vi "Read_CAL_PARAMETER_Connector_A.vi"() -> ()   [LabVIEW 2016]
doc: "The myRIO Project template acquires acceleration data from the onboard accelerometer and displays the changes of acceleration values in a waveform chart."
panel:
  in  "Tab Control":T1(tab)
  out "Device_ID 2":u8[](array[numeric]) format="%.0x"
  out "READ LSB CAL_PARAM 2":u8[][](array[numeric]) format="%.0x"
  out "READ MSB CAL_PARAM 2":u8[][](array[numeric]) format="%.0x"
  out "Array 3":i16[][](array[numeric])
  out "UT_Value 2":u16[](array[numeric])
  out "Temperature(°C)":dbl
  out "Waveform Chart Temperature":dbl(graph)
  out "Waveform Chart Presssure":dbl(graph)
  out "Pressure in Pa.":dbl
  out "error out 2":errorcluster
  out "UP_Value":u16[](array[numeric])
  # "Device is connceted to MXI connector A of the myRIO"
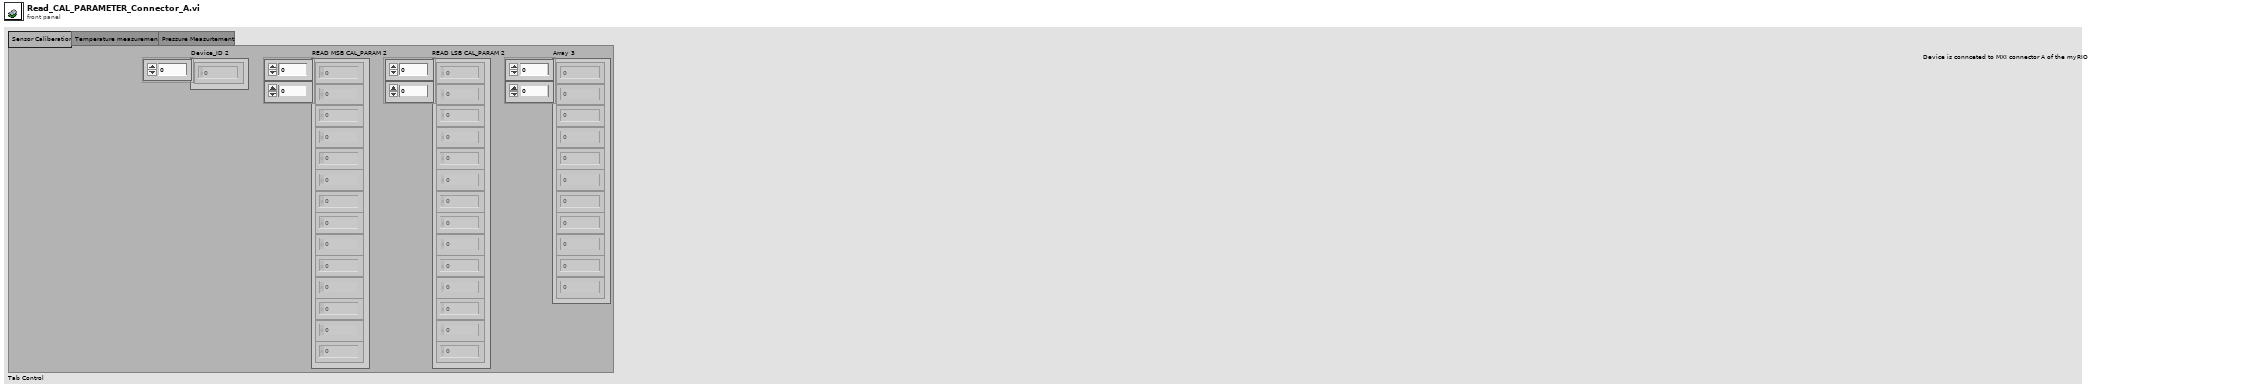
[diagram p1: front panel]
types:
  T1 = enum32{"Sensor Caliberation", "Temperature measurement", "Pressure Measurtement"}
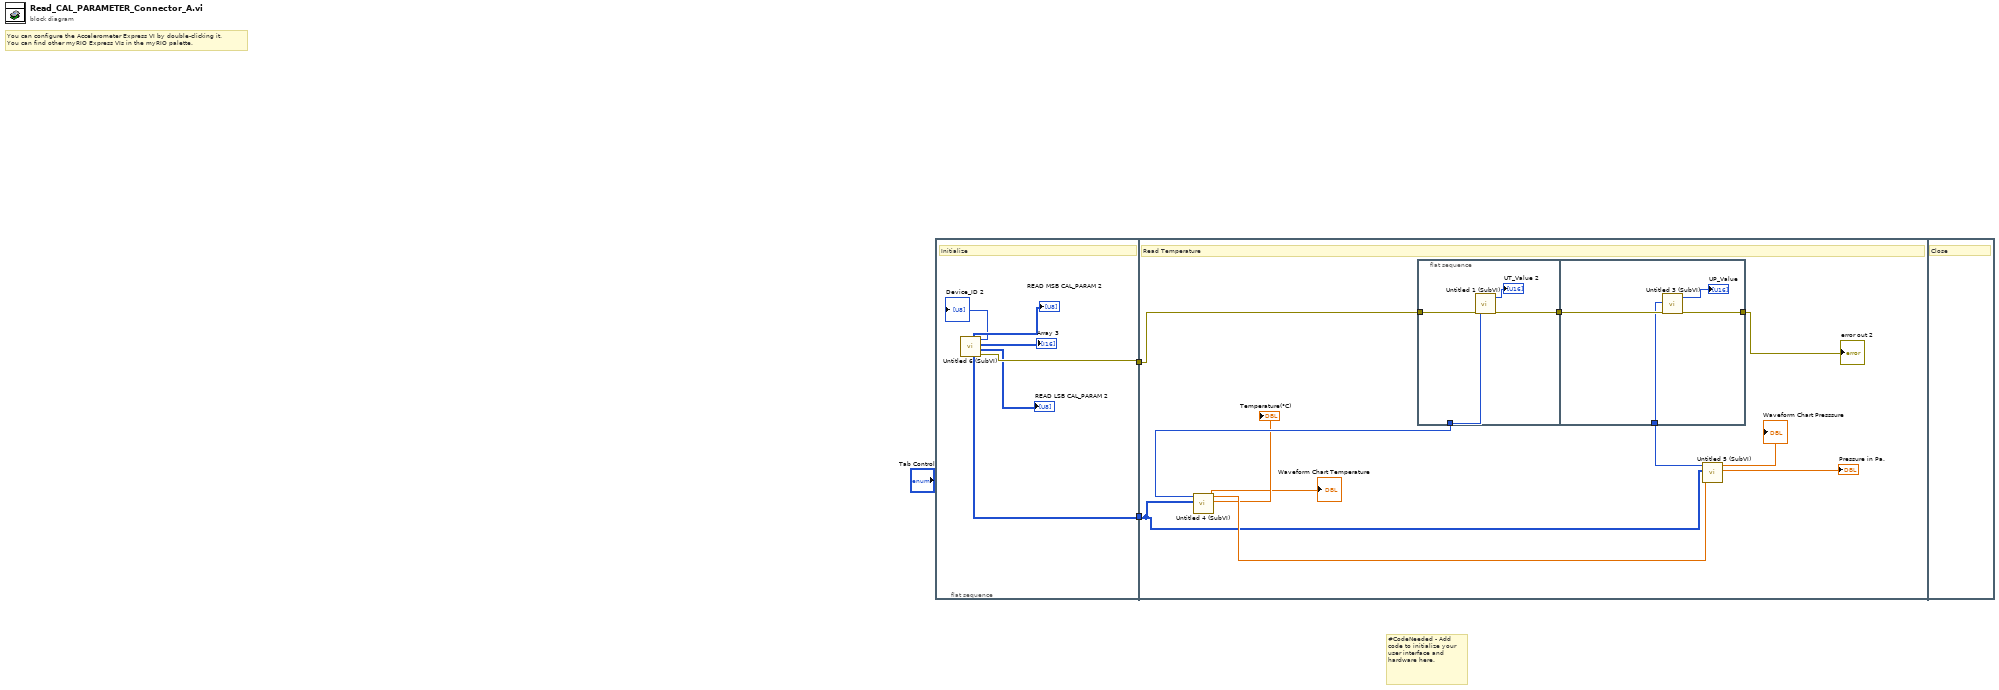
[diagram p0: block diagram]
diagram:
  # "#CodeNeeded - Add code to initialize your user interface and hardware here."
  # "You can configure the Accelerometer Express VI by double-clicking it.\nYou can find other myRIO Express VIs in the myRIO palette."
  n1 = flat-sequence {
    tunnel: [w8] -> w2
    tunnel: [w7] -> w1
    tunnel: w2 -> [w10]
    tunnel: w1 -> [w11]
    frame #0 {
      # "Initialize"
      n2 = call "Untitled 6 (SubVI).vi"() -> ("error out"=w8:errorcluster, "READ LSB CAL_PARAM 2"=→"READ LSB CAL_PARAM 2":u8[][], "Array 3"=→"Array 3":i16[][], "Device_ID 2"=→"Device_ID 2":u8[], "Array"=w7:u16[][], "READ MSB CAL_PARAM 2"=→"READ MSB CAL_PARAM 2":u8[][])  [unwired: 6 in]
    }
    frame #1 {
      # "Read Temperature"
      n3 = call "Untitled 4 (SubVI).vi"("Array"=w11, "Array 2"=w17) -> ("Waveform Chart"=→"Waveform Chart Temperature":dbl, "Temperature(°C)"=→"Temperature(°C)":dbl, "Numeric"=w16:dbl)  [unwired: 7 in]
      n4 = flat-sequence {
        tunnel: w10 -> [w23]
        tunnel: [w22] -> w19
        tunnel: [w21] -> w17
        tunnel: [w26] -> w18
        tunnel: w19 -> [w27]
        tunnel: [w25] -> w15
        frame #0 {
          n5 = call "Untitled 1 (SubVI).vi"("error in (no error)"=w23) -> ("error out"=w22:errorcluster, "Array"=w21:u16[], "UT_Value 2"=→"UT_Value 2":u16[])  [unwired: 8 in]
        }
        frame #1 {
          n6 = call "Untitled 3 (SubVI).vi"("error in (no error)"=w27) -> ("error out"=w26:errorcluster, "Array"=w25:u16[], "UP_Value"=→"UP_Value":u16[])  [unwired: 8 in]
        }
      }
      n7 = call "Untitled 5 (SubVI).vi"("Numeric"=w16, "Array"=w11, "Array 2"=w15) -> ("Pressure in Pa."=→"Pressure in Pa.":dbl, "Waveform Chart 2"=→"Waveform Chart Presssure":dbl)  [unwired: 7 in]
      "error out 2" <- w18
    }
    frame #2 {
      # "Close"
    }
  }
